vi "Login.vi"() -> (2 "Access":bool)   [LabVIEW 2013]
doc: "This VI is the solution to Exercise 3-1 of the LabVIEW Basics II course.\n\nThis VI will accept a user name and password, and after the OK button is pressed, verify if the information is valid using the Verify Information subVI. The name and password controls are initialized to empty strings and the Key Focus attribute of the Login Name control is set to TRUE.\n\nYou will use this VI in Application Exercise.vi (Exercise 5-1) as your login screen."
panel:
  in  "Cancle":bool
  in  "Ok":bool
  in  "Password":string
  in  "Login Name":string
  # "用户登录"
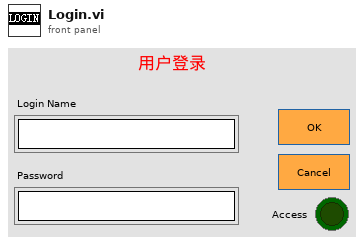
[diagram p1: front panel]
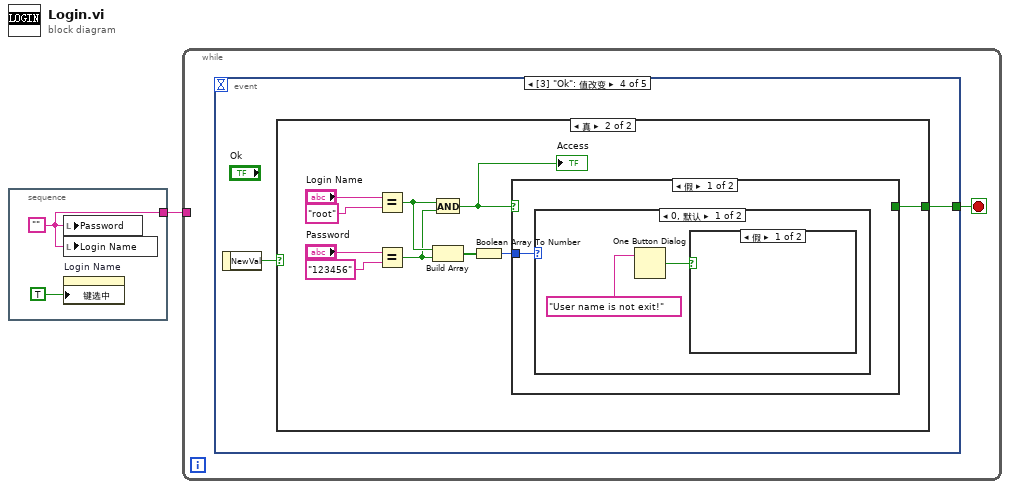
[diagram p0: block diagram]
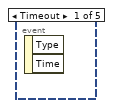
[diagram p2: hidden frame]
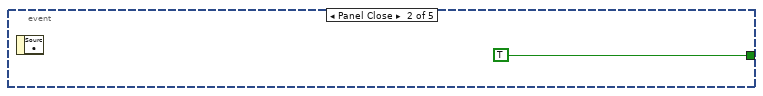
[diagram p3: hidden frame]
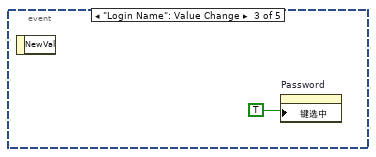
[diagram p4: hidden frame]
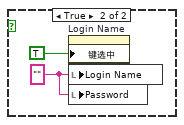
[diagram p6: hidden frame]
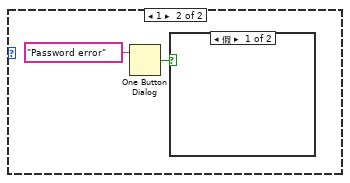
[diagram p7: hidden frame]
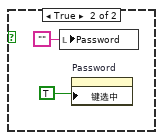
[diagram p8: hidden frame]
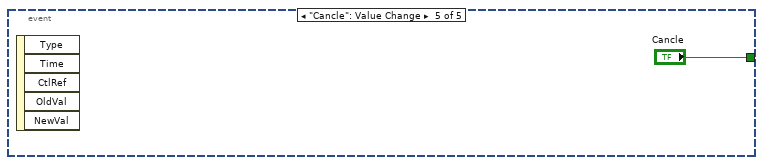
[diagram p10: hidden frame]
diagram:
  n1 = stacked-sequence {
    tunnel: [w2] -> w1
    frame #0 {
      w2 = ""
      n2 = local write "Password"(w2) -> ()
      n3 = local write "Login Name"(w2) -> ()
      n4 = property on="Login Name" class="Str"("键选中"=TRUE ("Key Focus")) -> ()  [unwired: 2 in, 2 out]
    }
  }
  n5 = while {
    tunnel: w1 -> [_]
    stop <- w4 stop-if-true
    n6 = event shown="[3] \"Ok\": 值改变" {
      selector: _ -> [_ _ _ _ _]
      dyn-events: _ -> [_ _ _ _ _]
      timeout: _ -> [_ _ _ _ _]
      tunnel: [_ TRUE ("Cancle") _ w7 "Cancle"] -> w4
      event Timeout {
        n7 = event-data() -> ()  [unwired: 3 out]
      }
      event Panel Close {
        n8 = event-data() -> ()  [unwired: 2 out]
      }
      event "Login Name": Value Change {
        n9 = event-data() -> ()  [unwired: 2 out]
        n10 = property on="Password" class="Str"("键选中"=TRUE ("Key Focus")) -> ()  [unwired: 2 in, 2 out]
      }
      event "Ok": Value Change {
        n11 = event-data() -> ("NewVal"=w8:bool)  [unwired: 1 out]
        n12 = case shown="真" w8 {
          tunnel: [_ w18] -> w7
          frame False {
          }
          frame True {
            n13 = Equal?(x="Login Name", y="root" ("User")) -> (x = y?=w14:bool)
            n14 = Equal?(x="Password", y="123456" ("ps")) -> (x = y?=w13:bool)
            n15 = And(x=w14, y=w13) -> (x .and. y?=w15:bool)
            "Access" <- w15
            n16 = Build Array(w14, w13) -> (w12:bool[])
            n17 = Boolean Array To Number(Boolean array=w12) -> (number=w11:u32)
            n18 = case shown="假" w15 {
              selector: w15 -> [_ w28]
              tunnel: [_ w28] -> w18
              tunnel: w11 -> [w19 _]
              frame False {
                n19 = case shown="0, 默认" w19 {
                  frame 0, Default {
                    n20 = One Button Dialog(message="User name is not exit!" ("消息")) -> (true=w20:bool)  [unwired: 1 out]
                    n21 = case shown="假" w20 {
                      frame False {
                      }
                      frame True {
                        w22 = "" ("Login Name")
                        n22 = property on="Login Name" class="Str"("键选中"=TRUE ("Key Focus")) -> ()  [unwired: 2 in, 2 out]
                        n23 = local write "Login Name"(w22) -> ()
                        n24 = local write "Password"(w22) -> ()
                      }
                    }
                  }
                  frame 1 {
                    n25 = One Button Dialog(message="Password error" ("消息")) -> (true=w24:bool)  [unwired: 1 out]
                    n26 = case shown="假" w24 {
                      frame False {
                      }
                      frame True {
                        n27 = local write "Password"("") -> ()
                        n28 = property on="Password" class="Str"("键选中"=TRUE ("Key Focus")) -> ()  [unwired: 2 in, 2 out]
                      }
                    }
                  }
                }
              }
              frame True {
              }
            }
          }
        }
      }
      event "Cancle": Value Change {
        n29 = event-data() -> ()  [unwired: 6 out]
      }
    }
  }
